vi "History Global.vi"() -> ()   [LabVIEW 2016, in "Path Track.lvlib"]
uses:
  Path Track.lvlib
panel:
  in  "Encoder R History":dbl[](array[numeric])
  in  "Encoder L History":dbl[](array[numeric])
  in  "Gyro History":dbl[](array[numeric])
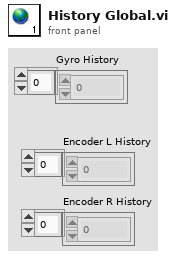
[diagram p1: front panel]
diagram:
